vi "Query PORT levels (scan).vi"(8 "error in (no error)":errorcluster, 10 "i (1)":i32=1, 11 "VISA resource name":refnum<visa-resource-name>) -> (0 "error out":errorcluster, 2 "output":dbl, 3 "VISA resource name out":refnum<visa-resource-name>)   [LabVIEW 2009, in "SR400.lvlib"]
doc: "PZ i\nThe PZ command returns the level of the PORT1\nand PORT2 outputs during a scan. i=1 or 2 to\nselect PORT1 or PORT 2 and is required. If the\nselected port is in the SCAN mode, its current\nlevel during a scan is read. If the counters are in\nreset or the output is in the FIXED mode, the PZ\ncommand returns the starting value for the level\n(same as PL command). The PZ command is a\nread only command."
uses:
  SR400.lvlib
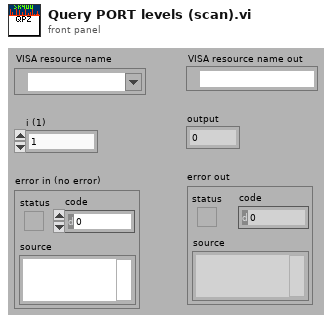
[diagram p1: front panel]
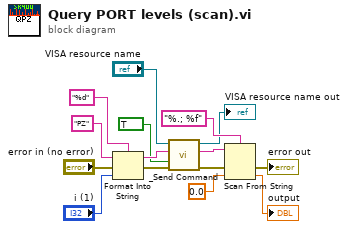
[diagram p0: block diagram]
diagram:
  n1 = Format Into String(format string="%d", initial string="PZ" ("command"), error in="error in (no error)", "i (1)") -> (resulting string=w6:string, error out=w5:errorcluster)
  n2 = call "_Send Command.vi"("error in (no error)"=w5, "Query? (F)"=TRUE, "Command"=w6, "VISA resource name"="VISA resource name") -> ("error out"=w2:errorcluster, "Response"=w3:string, "VISA resource name out"=→"VISA resource name out":refnum<visa-resource-name>)  [unwired: 5 out]
  n3 = Scan From String(format string="%.; %f", input string=w3, error in=w2, default 1=0.0 ("default value 1")) -> (error out=→"error out":errorcluster, output 1=→"output":dbl)  [unwired: 1 in, 2 out]
